vi "Pay.vi"(8 "error in (no error)":errorcluster, 10 "Amount":dbl, 11 "MonthlyExpense in":refnum<class "MonthlyExpense.lvclass">) -> (0 "error out":errorcluster, 2 "Balance":dbl, 3 "MonthlyExpense out":refnum<class "MonthlyExpense.lvclass">)   [LabVIEW 2020, in "MonthlyExpense.lvclass"]
uses:
  MonthlyExpense.lvclass
  MonthlyExpense.lvclass/MonthlyExpense.ctl
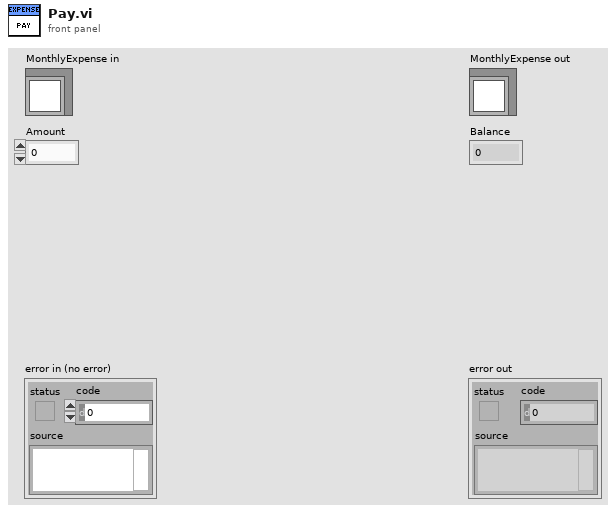
[diagram p1: front panel]
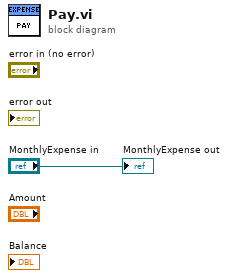
[diagram p0: block diagram]
diagram:
  "MonthlyExpense out" <- "MonthlyExpense in"
